vi "__Create New Bucket Dialog.vi"() -> ()   [LabVIEW 2011]
doc: "This is a pop-up dialog for creating a new bucket."
uses:
  vi.lib/National Instruments/LabVIEW Interface for Amazon S3/Typedefs/AMZ_S3_LocationConstraint.ctl
  vi.lib/National Instruments/LabVIEW Interface for Amazon S3/Typedefs/AMZ_S3_API_PUT Bucket Request Parameters.ctl
  vi.lib/National Instruments/LabVIEW Interface for Amazon S3/Typedefs/AMZ_S3_ACL.ctl
  vi.lib/National Instruments/LabVIEW Interface for Amazon S3/LV Interface for Amazon S3.lvlib
panel:
  in  "stop":bool
  in  "Create":bool
  in  "Bucket name":string
  in  "Location":T1=enum."EU"
  in  "Random":bool
  # "If you want to make a bucket in Amazon's default, US Classic region, you have to create it using another method!\nGo to \"https://console.aws.amazon.com/s3/home\" to access the AWS Console, where you can create the bucket."
  # "1. You can modify the Location to create the bucket in another Region\n2. Fill in a Bucket name, or Press Random name button any number of times to generate random names\n\n!!! The bucket name has to be globally unique !!!\n\n3. Press Create button to Create the bucket"
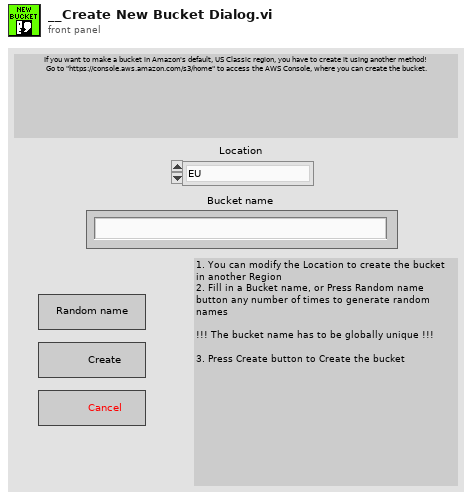
[diagram p1: front panel]
types:
  T1 = typedef "LV Interface for Amazon S3.lvlib/AMZ_S3_LocationConstraint.ctl" = enum16{"US Classic", "EU", "US-West-1", "AP-SouthEast-1"}
  T2 = typedef "LV Interface for Amazon S3.lvlib/AMZ_S3_API_PUT Bucket Request Parameters.ctl" = cluster{"ACL":T3, "Location":T1}
  T3 = typedef "LV Interface for Amazon S3.lvlib/AMZ_S3_ACL.ctl" = enum16{"private", "public-read", "public-read-write", "authenticated-read", "bucket-owner-read", "bucket-owner-full-control"}
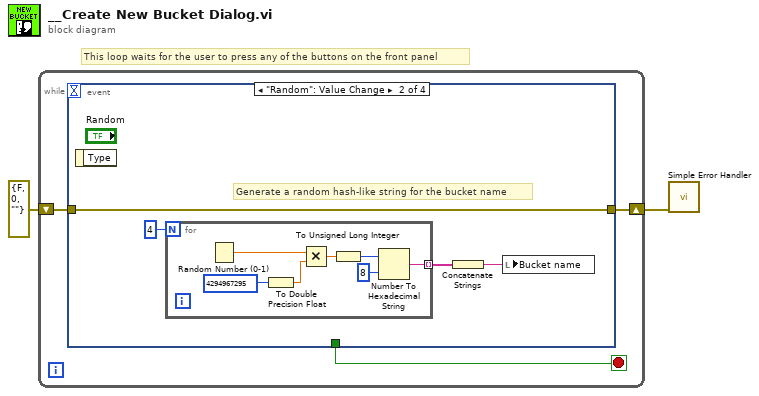
[diagram p0: block diagram]
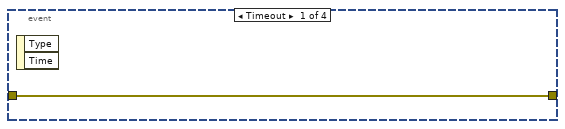
[diagram p2: hidden frame]
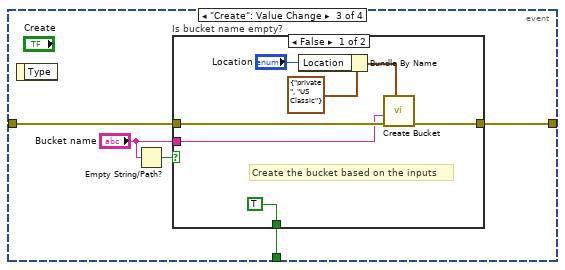
[diagram p3: hidden frame]
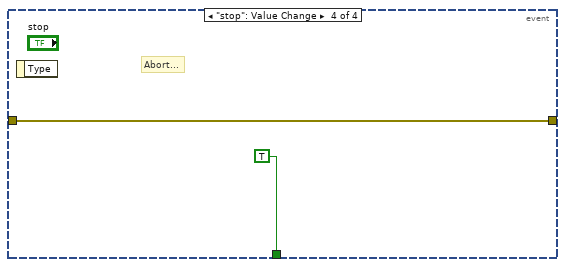
[diagram p5: hidden frame]
diagram:
  # "This loop waits for the user to press any of the buttons on the front panel"
  n1 = while {
    shift-right: [w3] -> w1
    shift-left: errorcluster {"status"=FALSE, "code"=0, "source"=""} ("error out") -> [w5]
    stop <- w4 stop-if-true
    n2 = event shown="[1] \"Random\": Value Change" {
      selector: _ -> [_ _ _ _]
      dyn-events: _ -> [_ _ _ _]
      timeout: _ -> [_ _ _ _]
      tunnel: w5 -> [w6 w8 w22 w31]
      tunnel: [_ _ w18 TRUE] -> w4
      tunnel: [w6 w8 w19 w31] -> w3
      event Timeout {
        n3 = event-data() -> ()  [unwired: 1 in, 2 out]
      }
      event "Random": Value Change {
        # "Generate a random hash-like string for the bucket name"
        n4 = event-data() -> ()  [unwired: 1 in, 1 out]
        n5 = for {
          N: 4 -> [_]
          tunnel: [w11] -> w9 mode=indexing
          n6 = Random Number (0-1)() -> (number: 0 to 1=w17:dbl)
          n7 = To Double Precision Float(number=u32 4294967295) -> (double precision float=w15:dbl)
          n8 = Multiply(x=w17, y=w15) -> (x*y=w14:dbl)
          n9 = To Unsigned Long Integer(number=w14) -> (unsigned 32bit integer=w13:u32)
          n10 = Number To Hexadecimal String(1:i16 8 ("width (-)"), 2:w13) -> (0:w11:string)
        }
        n11 = Concatenate Strings(w9) -> (w7:string)
        n12 = local write "Bucket name"(w7) -> ()
      }
      event "Create": Value Change {
        n13 = event-data() -> ()  [unwired: 1 in, 1 out]
        n14 = Empty String/Path?(string/path="Bucket name") -> (empty?=w21:bool)
        n15 = case "Is bucket name empty?" shown="False" w21 {
          tunnel: w22 -> [w27 w30]
          tunnel: "Bucket name" -> [w26 _]
          tunnel: [w24 w30] -> w19
          tunnel: [TRUE _] -> w18
          frame False {
            # "Create the bucket based on the inputs"
            n16 = Bundle By Name(cluster=T2 {"ACL"=enum."private", "Location"=enum."US Classic"} ("Request parameters"), "Location"="Location") -> (w25:T2)
            n17 = call "Create Bucket.vi"("Request parameters"=w25, "error in (no error)"=w27, "Bucket"=w26) -> ("error out"=w24:errorcluster)  [unwired: 8 in]
          }
          frame True {
          }
        }
      }
      event "stop": Value Change {
        # "Abort..."
        n18 = event-data() -> ()  [unwired: 1 in, 1 out]
      }
    }
  }
  n19 = call <vilib>:"Simple Error Handler.vi"("error in (no error)"=w1) -> ()  [unwired: 4 in, 5 out]
